vi "Write to Buffer.vi"(8 "error in (no error)":errorcluster, 10 "Data in":dbl[](array[numeric]), 11 "Waveform Receive in":refnum<class "Waveform Receive.lvclass">) -> (0 "error out":errorcluster, 3 "Waveform Receive out":refnum<class "Waveform Receive.lvclass">)   [LabVIEW 2012, in "Waveform Data Logger Engine.lvlib" / "Waveform Receive.lvclass"]
uses:
  Waveform Receive.lvclass
  Waveform Receive.lvclass/Waveform Receive.ctl
  Buffer/Waveform Buffer/Waveform Buffer.lvclass/Waveform Buffer.ctl
  Buffer/DBL Waveform Buffer/DBL Waveform Buffer.lvclass/DBL Waveform Buffer.ctl
  Buffer/Waveform Buffer/Update Current Segment.vi
  Buffer/Waveform Buffer/Check New Segment.vi
  Buffer/Waveform Buffer/Update Waveform Segments.vi
  Buffer/Waveform Buffer/Resize Buffer.vi
  Check For DBL Equality.vi
  Buffer/Waveform Buffer/Get Current Buffer Index.vi
  Buffer/Waveform Buffer/Get Buffer Length.vi
  Buffer/Waveform Buffer/Shift Point by Samples.vi
  Buffer/DBL Waveform Buffer/DBL Resize Buffer.vi
  Buffer/DBL Waveform Buffer/DBL Waveform Buffer.lvclass
  Buffer/CDB Waveform Buffer/CDB Waveform Buffer.lvclass
  Buffer/Waveform Buffer/Waveform Buffer.lvclass
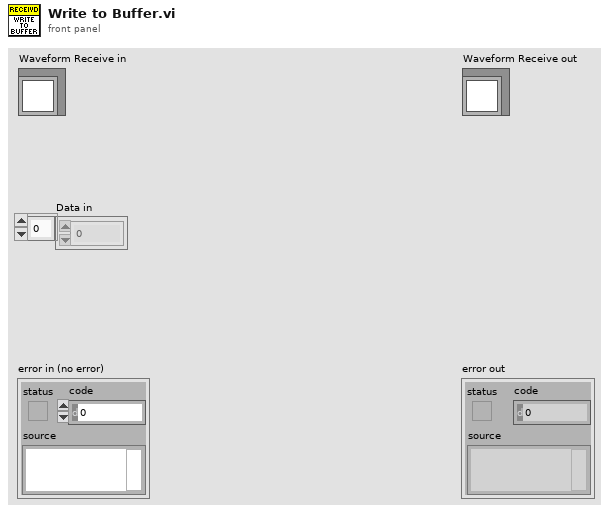
[diagram p1: front panel]
types:
  T1 = typedef "Waveform Data Logger Engine.lvlib/Waveform Receive.lvclass/Wfm Info.ctl" = cluster{"Segment ID":u64, "Size":i32, "dt":dbl, "t0":timestamp, "offset":u64, "receive time":timestamp}
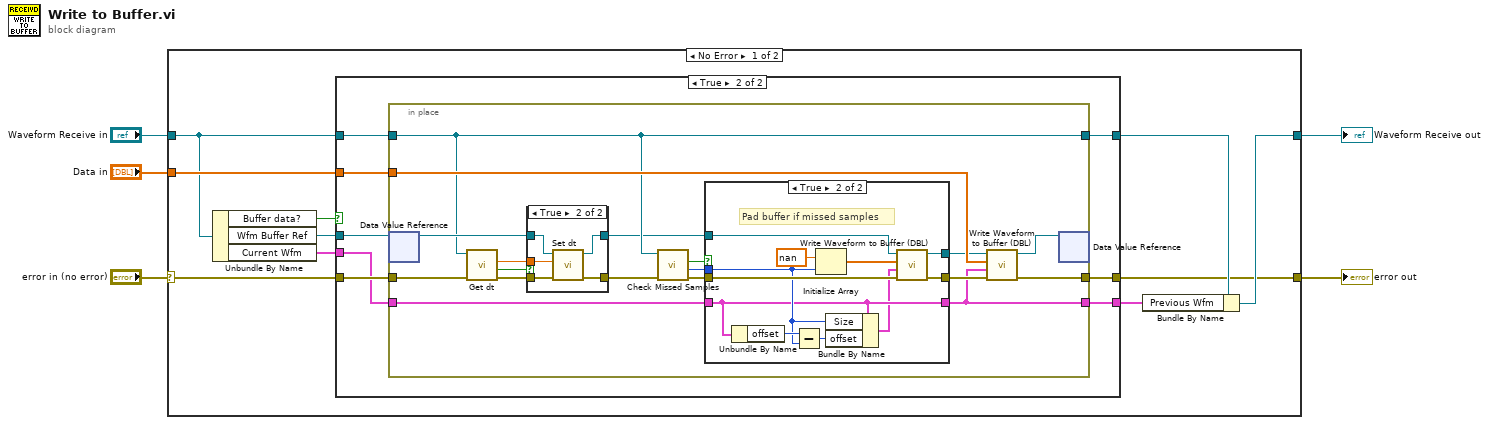
[diagram p0: block diagram]
diagram:
  n1 = case shown="No Error" "error in (no error)" {
    selector: "error in (no error)" -> [w15 w67]
    tunnel: [w7 w67] -> w4
    tunnel: [w8 w66] -> w3
    tunnel: "Waveform Receive in" -> [w12 w66]
    tunnel: "Data in" -> [w14 _]
    frame No Error {
      n2 = Unbundle By Name(w12) -> ("Buffer data?"=w6:bool, "Wfm Buffer Ref"=w13:refnum<data-value>, "Current Wfm"=w11:T1)
      n3 = case shown="True" w6 {
        tunnel: w15 -> [w17 w26]
        tunnel: w14 -> [_ w25]
        tunnel: w13 -> [_ w24]
        tunnel: w12 -> [w16 w23]
        tunnel: w11 -> [w18 w22]
        tunnel: [w16 w21] -> w10
        tunnel: [w18 w20] -> w9
        tunnel: [w17 w19] -> w7
        frame False {
        }
        frame True {
          n4 = in-place {
            in-place-border: w26 -> [w41]
            in-place-border: [w44] -> w19
            in-place-border: w25 -> [w43]
            in-place-border: w23 -> [w36]
            in-place-border: [w36] -> w21
            in-place-border: w22 -> [w28]
            in-place-border: [w27] -> w20
            n5 = in-place-dvr #1(w24) -> (w42:refnum<class "Waveform Buffer.lvclass">)  [unwired: 1 out]
            n6 = call "Get dt.vi"("error in (no error)"=w41, "Waveform Receive in"=w36) -> ("error out"=w38:errorcluster, "dt Changed?"=w39:bool, "dt"=w40:dbl)  [unwired: 6 in, 1 out]
            n7 = case shown="True" w39 {
              tunnel: w42 -> [w60 w65]
              tunnel: [w60 w64] -> w34
              tunnel: [w59 w63] -> w37
              tunnel: w38 -> [w59 w62]
              tunnel: w40 -> [_ w61]
              frame False {
              }
              frame True {
                n8 = call "Set dt.vi"("error in (no error)"=w62, "dt"=w61, "Waveform Buffer in"=w65) -> ("error out"=w63:errorcluster, "Waveform Buffer out"=w64:refnum<class "Waveform Buffer.lvclass">)  [unwired: 7 in]
              }
            }
            n9 = call "Check Missed Samples.vi"("error in (no error)"=w37, "Waveform Receive in"=w36) -> ("error out"=w35:errorcluster, "Samples Missed"=w29:u64, "Missing Samples?"=w30:bool)  [unwired: 6 in, 1 out]
            n10 = case shown="True" w30 {
              tunnel: w35 -> [w46 w55]
              tunnel: w34 -> [w47 w57]
              tunnel: w28 -> [w45 w49]
              tunnel: [w47 w54] -> w33
              tunnel: [w46 w53] -> w31
              tunnel: w29 -> [_ w50]
              tunnel: [w45 w49] -> w27
              frame False {
              }
              frame True {
                # "Pad buffer if missed samples"
                n11 = Unbundle By Name(w49) -> ("offset"=w52:u64)
                n12 = Subtract(x=w52, y=w50) -> (x-y=w51:u64)
                n13 = Initialize Array(nan, w50) -> (w56:dbl[])
                n14 = Bundle By Name(cluster=w49, "Size"=w50, "offset"=w51) -> (w48:T1)
                n15 = call "Write Waveform to Buffer (DBL).vi"("error in (no error)"=w55, "Waveform Info"=w48, "Data"=w56, "Waveform Buffer in"=w57) -> ("error out"=w53:errorcluster, "Waveform Buffer out"=w54:refnum<class "Waveform Buffer.lvclass">)  [unwired: 6 in]
              }
            }
            n16 = call "Write Waveform to Buffer (DBL).vi"("error in (no error)"=w31, "Waveform Info"=w27, "Data"=w43, "Waveform Buffer in"=w33) -> ("error out"=w44:errorcluster, "Waveform Buffer out"=w32:refnum<class "Waveform Buffer.lvclass">)  [unwired: 6 in]
            n17 = in-place-dvr #1(w32) -> ()  [unwired: 2 out]
          }
        }
      }
      n18 = Bundle By Name(cluster=w10, "Previous Wfm"=w9) -> (w8:refnum<class "Waveform Receive.lvclass">)
    }
    frame Error {
    }
  }
  "error out" <- w4
  "Waveform Receive out" <- w3
